vi "fileNamePrefix.vi"(10 "Bank":i32, 11 "Index":i32) -> (3 "Prefix String":string)   [LabVIEW 2019]
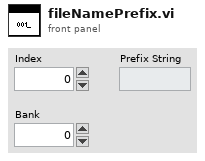
[diagram p1: front panel]
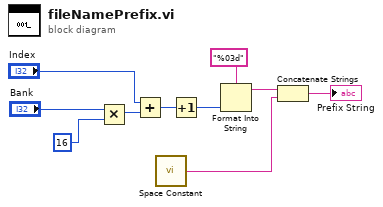
[diagram p0: block diagram]
diagram:
  n1 = Multiply(x="Bank", y=16) -> (x*y=w7:i32)
  n2 = Add(x="Index", y=w7) -> (x+y=w6:i32)
  n3 = call <vilib>:"Space Constant.vi"() -> ("String"=w4:string)
  n4 = Increment(x=w6) -> (x+1=w3:i32)
  n5 = Format Into String(format string="%03d", w3) -> (resulting string=w1:string)  [unwired: 2 in, 1 out]
  n6 = Concatenate Strings(w1, w4) -> (→"Prefix String":string)
